vi "Consumer.vi"(8 "error in (no error)":errorcluster, 9 "Data":variant, 10 "Case ID":string, 11 "uService Template in":refnum<class "Test_uService.lvclass">) -> (0 "error out":errorcluster, 3 "uService Template out":refnum<class "Test_uService.lvclass">)   [LabVIEW 2020, in "Test_uService.lvlib" / "Test_uService.lvclass"]
uses:
  Test_uService.lvclass
  Test_uService Consumer Case Selector.ctl
  <vilib>/Analysis/NI_AALBase.lvlib
  TALOS/TALOS_PPL.lvlibp/Father of all uServices/Father of all uServices/Father of all uServices.lvclass
  C:/LabVIEW Code/aegis-labview-code/TALOS/TALOS_PPL.lvlibp/Father of all uServices/Father of all uServices/Father of all uServices.lvclass
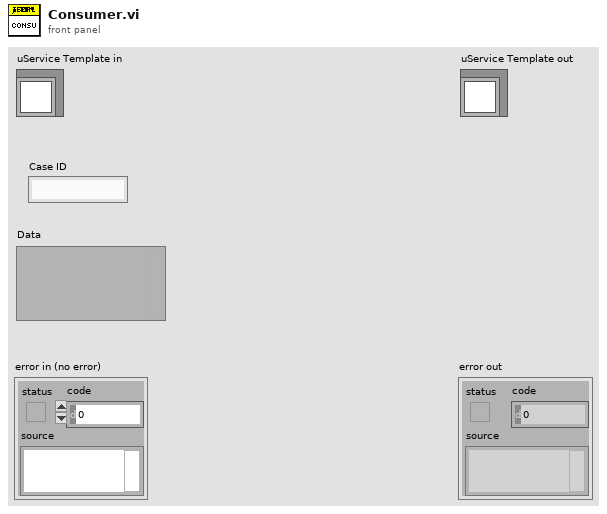
[diagram p1: front panel]
types:
  T1 = typedef "Test_uService.lvlib/Test_uService.lvclass/Test_uService Consumer Case Selector.ctl" = enum16{"Start echo", "Echo arrived"}
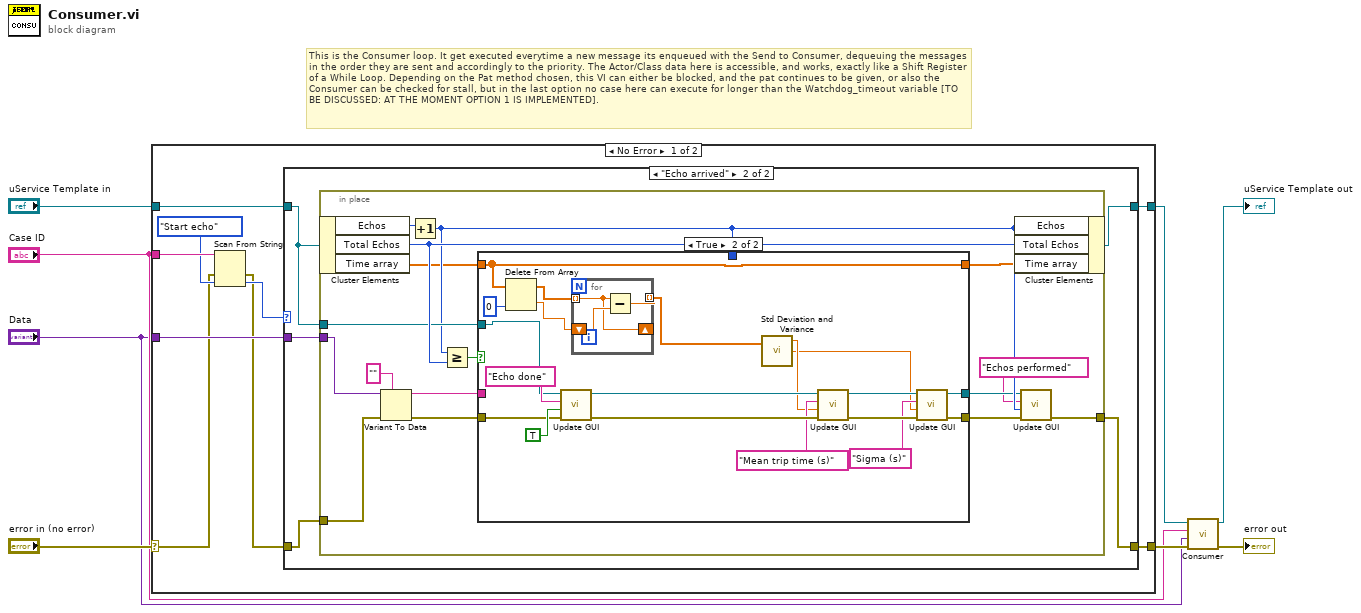
[diagram p0: block diagram]
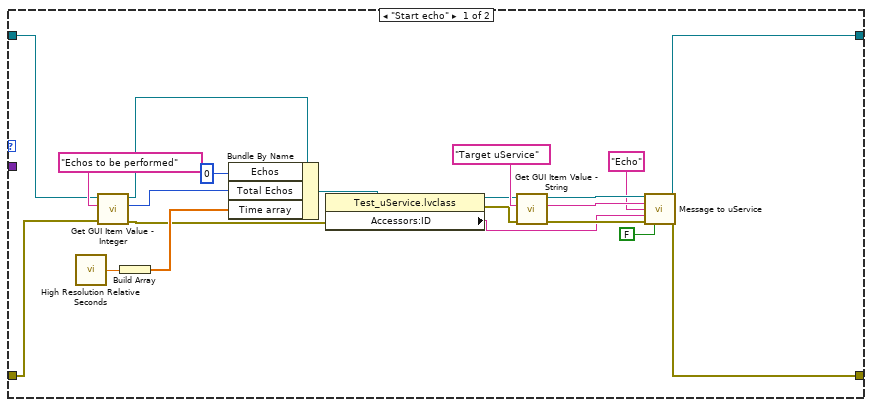
[diagram p2: hidden frame]
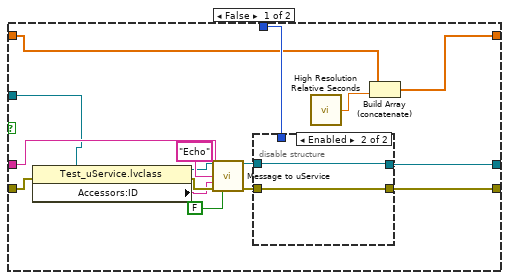
[diagram p3: hidden frame]
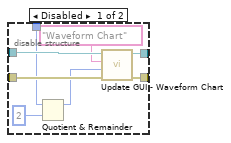
[diagram p4: hidden frame]
diagram:
  # "This is the Consumer loop. It get executed everytime a new message its enqueued with the Send to Consumer, dequeuing the messages in the order they are sent and accordingly to the priority. The Actor/Class data here is accessible, and works, exactly like a Shift Register of a While Loop. Depending on the Pat method chosen, this VI can either be blocked, and the pat continues to be given, or also the Consumer can be checked for stall, but in the last option no case here can execute for longer than the Watchdog_timeout variable [TO BE DISCUSSED: AT THE MOMENT OPTION 1 IS IMPLEMENTED]."
  n1 = case shown="No Error" "error in (no error)" {
    selector: "error in (no error)" -> [w11 w108]
    tunnel: [w16 w109] -> w3
    tunnel: "uService Template in" -> [w17 w109]
    tunnel: [w9 w108] -> w6
    tunnel: "Case ID" -> [w14 _]
    tunnel: "Data" -> [w15 _]
    frame No Error {
      n2 = Scan From String(input string=w14, error in=w11, default 1=Test_uService_Consumer_Case_Selector."Start echo" ("Consumer Case Selector")) -> (error out=w10:errorcluster, output 1=w12:T1)  [unwired: 2 in, 2 out]
      n3 = case shown="\"Echo arrived\"" w12 {
        tunnel: w17 -> [w34 w40]
        tunnel: [w29 w42] -> w16
        tunnel: w15 -> [_ w41]
        tunnel: w10 -> [w36 w43]
        tunnel: [w27 w39] -> w9
        frame "Start echo" {
          n4 = call <vilib>:"High Resolution Relative Seconds.vi"() -> ("relative seconds"=w26:dbl)
          n5 = call "Get GUI Item Value - Integer.vi"("error in (no error)"=w36, "FP Item Name"="Echos to be performed", "uService Template in"=w34) -> ("error out"=w21:errorcluster, "Value"=w33:i32, "uService Template out"=w35:refnum<class "Test_uService.lvclass">)  [unwired: 6 in]
          n6 = Build Array(w26) -> (w25:dbl[])
          n7 = Bundle By Name(cluster=w35, "Echos"=u16 0, "Total Echos"=w33, "Time array"=w25) -> (w23:refnum<class "Test_uService.lvclass">)
          n8 = property class="Test_uService.lvclass"(reference=w23, error in=w21) -> (reference out=w22:refnum<class "Test_uService.lvclass">, error out=w20:errorcluster, "Accessors:ID"=w19:string)
          n9 = call "Get GUI Item Value - String.vi"("error in (no error)"=w20, "FP Item Name"="Target uService", "uService Template in"=w22) -> ("error out"=w28:errorcluster, "Value"=w31:string, "uService Template out"=w30:refnum<class "Test_uService.lvclass">)  [unwired: 6 in]
          n10 = call "Message to uService.vi"("Father of all uServices in"=w30, "uService ID"=w31, "Message"="Echo" ("Item Name"), "Data"=w19, "error in (no error)"=w28, "Locale?"=FALSE) -> ("Father of all uServices out"=w29:refnum<class "Test_uService.lvclass">, "error out"=w27:errorcluster)  [unwired: 8 in]
        }
        frame "Echo arrived" {
          n11 = in-place {
            in-place-border: w43 -> [w56]
            in-place-border: w41 -> [w58]
            in-place-border: w40 -> [w51]
            in-place-border: [w49] -> w39
            n12 = in-place-cluster #1(w40) -> ("Echos"=w59:u16, "Total Echos"=w55:u16, "Time array"=w45:dbl[])
            n13 = Variant To Data(error in=w56, type="" ("Item Name"), Variant=w58) -> (data=w53:string, error out=w52:errorcluster)
            n14 = Increment(x=w59) -> (x+1=w48:u16)
            n15 = Greater Or Equal?(x=w48, y=w55) -> (x >= y?=w54:bool)
            n16 = case shown="True" w54 {
              tunnel: w53 -> [w75 _]
              tunnel: w52 -> [w63 w102]
              tunnel: w51 -> [w64 w101]
              tunnel: [w72 w94] -> w50
              tunnel: w48 -> [w71 _]
              tunnel: [w70 w95] -> w47
              tunnel: w45 -> [w69 w90]
              tunnel: [w68 w90] -> w44
              frame False {
                n17 = property class="Test_uService.lvclass"(reference=w64, error in=w63) -> (reference out=w65:refnum<class "Test_uService.lvclass">, error out=w62:errorcluster, "Accessors:ID"=w61:string)
                n18 = call "Message to uService.vi"("Father of all uServices in"=w65, "uService ID"=w75, "Message"="Echo" ("Item Name"), "Data"=w61, "error in (no error)"=w62, "Locale?"=FALSE) -> ("Father of all uServices out"=w73:refnum<class "Test_uService.lvclass">, "error out"=w74:errorcluster)  [unwired: 8 in]
                n19 = disable-structure shown="Enabled" {
                  disable-tunnel: w74 -> [w83 w84]
                  disable-tunnel: w73 -> [w82 w85]
                  disable-tunnel: [w81 w84] -> w72
                  disable-tunnel: w71 -> [w79 _]
                  disable-tunnel: [w76 w85] -> w70
                  frame Disabled {
                    n20 = Quotient & Remainder(x=w79, y=u16 2) -> (x-y*floor(x/y)=w77:u16)  [unwired: 1 out]
                    n21 = call "Update GUI - Waveform Chart.vi"("error in (no error)"=w83, "Point value"=w77, "GUI Item Name"="Waveform Chart", "uService Template in"=w82) -> ("error out"=w81:errorcluster, "uService Template out"=w76:refnum<class "Test_uService.lvclass">)  [unwired: 6 in]
                  }
                  frame Enabled {
                  }
                }
                n22 = call <vilib>:"High Resolution Relative Seconds.vi"() -> ("relative seconds"=w67:dbl)
                n23 = Build Array (concatenate)(w69, w67) -> (w68:dbl[])
              }
              frame True {
                n24 = Delete From Array(array=w90, index=0) -> (deleted portion=w87:dbl, array with subset deleted=w88:dbl[])  [unwired: 1 in]
                n25 = call "Update GUI.vi"("error in (no error)"=w102, "Data"=TRUE, "GUI Item Name"="Echo done", "uService Template in"=w101) -> ("error out"=w99:errorcluster, "uService Template out"=w100:refnum<class "Test_uService.lvclass">)  [unwired: 6 in]
                n26 = for {
                  tunnel: w88 -> [w105] mode=indexing
                  shift-right: [w105] -> _
                  shift-left: w87 -> [w107]
                  tunnel: [w106] -> w86 mode=indexing
                  n27 = Subtract(x=w105, y=w107) -> (x-y=w106:dbl)
                }
                n28 = call <vilib>:"Std Deviation and Variance.vi"("X"=w86) -> ("mean"=w92:dbl, "standard deviation"=w91:dbl)  [unwired: 1 in, 1 out]
                n29 = call "Update GUI.vi"("error in (no error)"=w99, "Data"=w92, "GUI Item Name"="Mean trip time (s)", "uService Template in"=w100) -> ("error out"=w96:errorcluster, "uService Template out"=w97:refnum<class "Test_uService.lvclass">)  [unwired: 6 in]
                n30 = call "Update GUI.vi"("error in (no error)"=w96, "Data"=w91, "GUI Item Name"="Sigma (s)", "uService Template in"=w97) -> ("error out"=w94:errorcluster, "uService Template out"=w95:refnum<class "Test_uService.lvclass">)  [unwired: 6 in]
              }
            }
            n31 = in-place-cluster #1("Echos"=w48, "Total Echos"=w55, "Time array"=w44) -> (w42:refnum<class "Test_uService.lvclass">)
            n32 = call "Update GUI.vi"("error in (no error)"=w50, "Data"=w48, "GUI Item Name"="Echos performed", "uService Template in"=w47) -> ("error out"=w49:errorcluster)  [unwired: 6 in, 1 out]
          }
        }
      }
    }
    frame Error {
    }
  }
  n33 = call-parent "Consumer.vi"("error in (no error)"=w6, "Data"="Data", "Case ID"="Case ID", "uService Template in"=w3) -> ("error out"=→"error out":errorcluster, "uService Template out"=→"uService Template out":refnum<class "Test_uService.lvclass">)  [unwired: 6 in]
